vi "Select Operation To send (SubVI).vi"(0 "Combo Box":string, 1 "POT":u16(ring) items=["X", "Y", "Z"], 2 "POT_Value":u16 format="%.0x", 3 "CheckSum":u32 format="%.0x", 4 "Ch XYZ":u8(ring) items=["Ch X", "Ch Y", "Ch Z"], 6 "Ch 3":u8(ring) items=["Ch X", "Ch Y", "Ch Z"], 7 "S/N":u8, 8 "SF A":i32, 10 "SF B":i32, 12 "SF C":i32) -> (16 "write":u8[](array[numeric]))   [LabVIEW 2017]
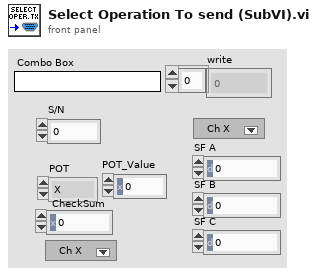
[diagram p1: front panel]
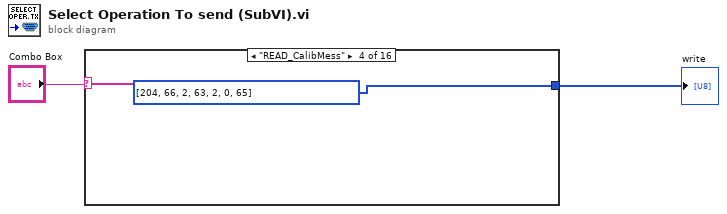
[diagram p0: block diagram]
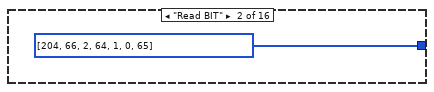
[diagram p3: hidden frame]
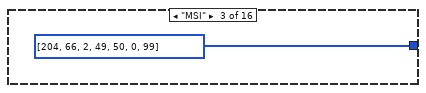
[diagram p4: hidden frame]
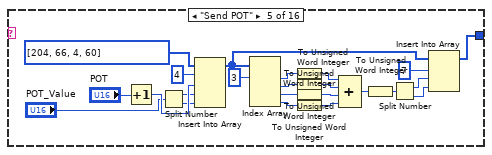
[diagram p5: hidden frame]
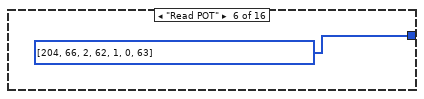
[diagram p6: hidden frame]
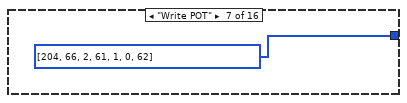
[diagram p7: hidden frame]
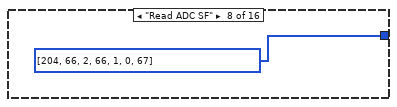
[diagram p8: hidden frame]
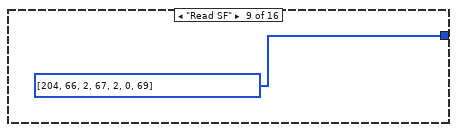
[diagram p9: hidden frame]
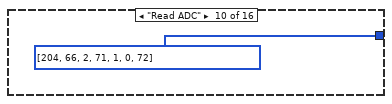
[diagram p10: hidden frame]
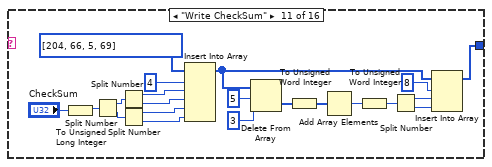
[diagram p11: hidden frame]
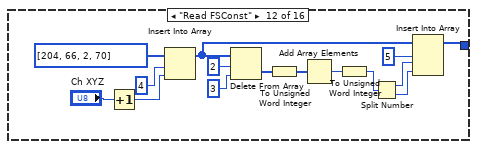
[diagram p12: hidden frame]
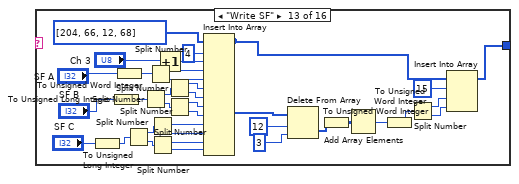
[diagram p13: hidden frame]
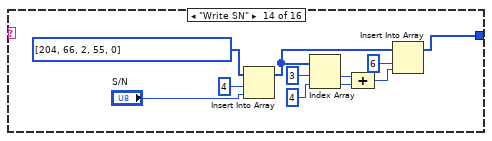
[diagram p14: hidden frame]
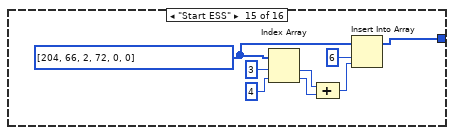
[diagram p15: hidden frame]
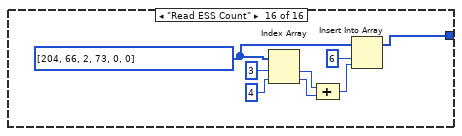
[diagram p16: hidden frame]
diagram:
  n1 = case shown="\"READ_CalibMess\"" "Combo Box" {
    tunnel: [_ u8[] [204, 66, 2, 64, 1, 0, 65] ("write") u8[] [204, 66, 2, 49, 50, 0, 99] ("write") u8[] [204, 66, 2, 63, 2, 0, 65] ("write") w6 u8[] [204, 66, 2, 62, 1, 0, 63] ("write") u8[] [204, 66, 2, 61, 1, 0, 62] ("write") u8[] [204, 66, 2, 66, 1, 0, 67] ("write") u8[] [204, 66, 2, 67, 2, 0, 69] ("write") u8[] [204, 66, 2, 71, 1, 0, 72] ("write") w34 w55 w71 w105 w116 w124] -> w1
    frame "", Default {
    }
    frame "Read BIT" {
    }
    frame "MSI" {
    }
    frame "READ_CalibMess" {
    }
    frame "Send POT" {
      n2 = Increment(x="POT") -> (x+1=w28:u16)
      n3 = Split Number(x="POT_Value") -> (hi(x)=w24:u8, lo(x)=w25:u8)
      n4 = Insert Into Array(array=u8[] [204, 66, 4, 60] ("write"), index=4, new element #1=w28, new element #2=w24, new element #3=w25) -> (w26:u8[])
      n5 = Index Array(array=w26, index #1=3) -> (element #1=w11:u8, element #2=w17:u8, element #3=w18:u8, element #4=w19:u8)  [unwired: 3 in]
      n6 = To Unsigned Word Integer(number=w11) -> (unsigned 16bit integer=w16:u16)
      n7 = To Unsigned Word Integer(number=w17) -> (unsigned 16bit integer=w15:u16)
      n8 = To Unsigned Word Integer(number=w18) -> (unsigned 16bit integer=w14:u16)
      n9 = To Unsigned Word Integer(number=w19) -> (unsigned 16bit integer=w13:u16)
      n10 = Compound Arithmetic op=ADD(w16, w15, w14, w13) -> (w12:u16)
      n11 = To Unsigned Word Integer(number=w12) -> (unsigned 16bit integer=w20:u16)
      n12 = Split Number(x=w20) -> (hi(x)=w21:u8, lo(x)=w22:u8)
      n13 = Insert Into Array(array=w26, index=7, new element #1=w21, new element #2=w22) -> (w6:u8[])
    }
    frame "Read POT" {
    }
    frame "Write POT" {
    }
    frame "Read ADC SF" {
    }
    frame "Read SF" {
    }
    frame "Read ADC" {
    }
    frame "Write CheckSum" {
      n14 = To Unsigned Long Integer(number="CheckSum") -> (unsigned 32bit integer=w54:u32)
      n15 = Split Number(x=w54) -> (hi(x)=w52:u16, lo(x)=w53:u16)
      n16 = Split Number(x=w52) -> (hi(x)=w50:u8, lo(x)=w49:u8)
      n17 = Split Number(x=w53) -> (hi(x)=w48:u8, lo(x)=w47:u8)
      n18 = Insert Into Array(array=u8[] [204, 66, 5, 69] ("write"), index=4, new element #1=w50, new element #2=w49, new element #3=w48, new element #4=w47) -> (w42:u8[])
      n19 = Delete From Array(array=w42, length=5, index=3) -> (deleted portion=w46:u8[])  [unwired: 1 out]
      n20 = To Unsigned Word Integer(number=w46) -> (unsigned 16bit integer=w45:u16[])
      n21 = Add Array Elements(numeric array=w45) -> (sum=w41:u16)
      n22 = To Unsigned Word Integer(number=w41) -> (unsigned 16bit integer=w40:u16)
      n23 = Split Number(x=w40) -> (hi(x)=w43:u8, lo(x)=w44:u8)
      n24 = Insert Into Array(array=w42, index=8, new element #1=w43, new element #2=w44) -> (w34:u8[])
    }
    frame "Read FSConst" {
      n25 = Increment(x="Ch XYZ") -> (x+1=w69:u8)
      n26 = Insert Into Array(array=u8[] [204, 66, 2, 70] ("write"), index=4, new element=w69) -> (w63:u8[])
      n27 = Delete From Array(array=w63, length=2, index=3) -> (deleted portion=w67:u8[])  [unwired: 1 out]
      n28 = To Unsigned Word Integer(number=w67) -> (unsigned 16bit integer=w66:u16[])
      n29 = Add Array Elements(numeric array=w66) -> (sum=w62:u16)
      n30 = To Unsigned Word Integer(number=w62) -> (unsigned 16bit integer=w61:u16)
      n31 = Split Number(x=w61) -> (hi(x)=w64:u8, lo(x)=w65:u8)
      n32 = Insert Into Array(array=w63, index=5, new element #1=w64, new element #2=w65) -> (w55:u8[])
    }
    frame "Write SF" {
      n33 = To Unsigned Long Integer(number="SF C") -> (unsigned 32bit integer=w84:u32)
      n34 = To Unsigned Long Integer(number="SF B") -> (unsigned 32bit integer=w83:u32)
      n35 = To Unsigned Word Integer(number="SF A") -> (unsigned 16bit integer=w89:u16)
      n36 = Split Number(x=w84) -> (hi(x)=w80:u16, lo(x)=w81:u16)
      n37 = Split Number(x=w83) -> (hi(x)=w78:u16, lo(x)=w77:u16)
      n38 = Split Number(x=w89) -> (hi(x)=w91:u8, lo(x)=w92:u8)
      n39 = Split Number(x=w80) -> (hi(x)=w97:u8, lo(x)=w98:u8)
      n40 = Split Number(x=w81) -> (hi(x)=w99:u8, lo(x)=w70:u8)
      n41 = Increment(x="Ch 3") -> (x+1=w100:u8)
      n42 = Split Number(x=w78) -> (hi(x)=w93:u8, lo(x)=w94:u8)
      n43 = Split Number(x=w77) -> (hi(x)=w95:u8, lo(x)=w96:u8)
      n44 = Insert Into Array(array=u8[] [204, 66, 12, 68] ("write"), index=4, new element #1=w100, new element #2=w91, new element #3=w92, new element #4=w93, new element #5=w94, new element #6=w95, new element #7=w96, new element #8=w97, new element #9=w98, new element #10=w99, new element #11=w70) -> (w102:u8[])
      n45 = Delete From Array(array=w102, length=12, index=3) -> (deleted portion=w85:u8[])  [unwired: 1 out]
      n46 = To Unsigned Word Integer(number=w85) -> (unsigned 16bit integer=w88:u16[])
      n47 = Add Array Elements(numeric array=w88) -> (sum=w86:u16)
      n48 = To Unsigned Word Integer(number=w86) -> (unsigned 16bit integer=w87:u16)
      n49 = Split Number(x=w87) -> (hi(x)=w103:u8, lo(x)=w104:u8)
      n50 = Insert Into Array(array=w102, index=15, new element #1=w103, new element #2=w104) -> (w71:u8[])
    }
    frame "Write SN" {
      n51 = Insert Into Array(array=u8[] [204, 66, 2, 55, 0] ("write"), index=4, new element="S/N") -> (w111:u8[])
      n52 = Index Array(array=w111, index #1=3, index #2=4) -> (element #1=w112:u8, element #2=w113:u8)
      n53 = Compound Arithmetic op=ADD(w112, w113) -> (w114:u8)
      n54 = Insert Into Array(array=w111, index=6, new element=w114) -> (w105:u8[])
    }
    frame "Start ESS" {
      w120 = u8[] [204, 66, 2, 72, 0, 0] ("write")
      n55 = Index Array(array=w120, index #1=3, index #2=4) -> (element #1=w121:u8, element #2=w122:u8)
      n56 = Compound Arithmetic op=unknown(w121, w122) -> (w123:u8)
      n57 = Insert Into Array(array=w120, index=6, new element=w123) -> (w116:u8[])
    }
    frame "Read ESS Count" {
      w128 = u8[] [204, 66, 2, 73, 0, 0] ("write")
      n58 = Index Array(array=w128, index #1=3, index #2=4) -> (element #1=w129:u8, element #2=w130:u8)
      n59 = Compound Arithmetic op=unknown(w129, w130) -> (w131:u8)
      n60 = Insert Into Array(array=w128, index=6, new element=w131) -> (w124:u8[])
    }
  }
  "write" <- w1
